vi "String Equals Ignore Case.vi"(0 "String":string, 1 "String 2":string) -> (3 "equal?":bool)   [LabVIEW 2023]
doc: "Compares two strings and declares them equal if they are the same characters, ignoring any case differences (as defined by the <b>To Lower Case</b> function). In other words, \"AbC\" is equal to \"aBc\"."
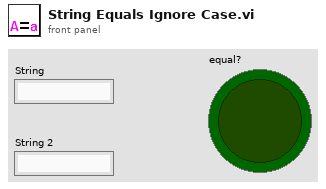
[diagram p1: front panel]
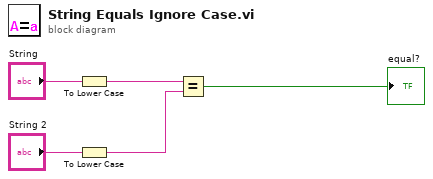
[diagram p0: block diagram]
diagram:
  n1 = To Lower Case(string="String") -> (all lower case string=w1:string)
  n2 = To Lower Case(string="String 2") -> (all lower case string=w4:string)
  n3 = Equal?(x=w1, y=w4) -> (x = y?=→"equal?":bool)
